vi "Get Tach Period (FPGA).vi"(9 "Threshold Settings":T1={"threshold"=0.0, "hysteresis"=0.0, "slope (rising)"=enum."rising"}, 10 "Max Tach Period (uSec)":u32=1000000, 11 "Analog Tach Signal":fxp<+/-,24,4>) -> (1 "Tach State":T2, 2 "Tach Period (uSec/pulse)":u32)   [LabVIEW 2014, in "Tachometer (SGL).lvlib"]
doc: "Convert analog tachometer signal to RPM"
uses:
  Tachometer (SGL).lvlib
  Tach State.ctl
  Threshold Settings.ctl
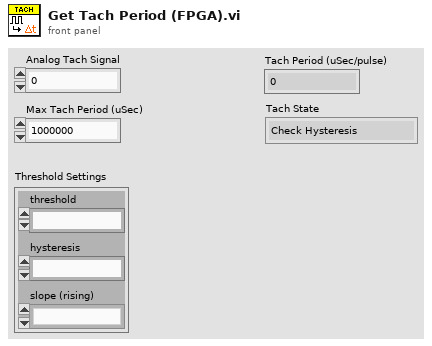
[diagram p1: front panel]
types:
  T1 = typedef "Tachometer (SGL).lvlib/Threshold Settings.ctl" = cluster{"threshold":fxp<+/-,24,4>, "hysteresis":fxp<+/-,24,4>, "slope (rising)":enum16{"falling", "rising"}}
  T2 = typedef "Tachometer (SGL).lvlib/Tach State.ctl" = enum16{"Check Hysteresis", "Check Threshold"}
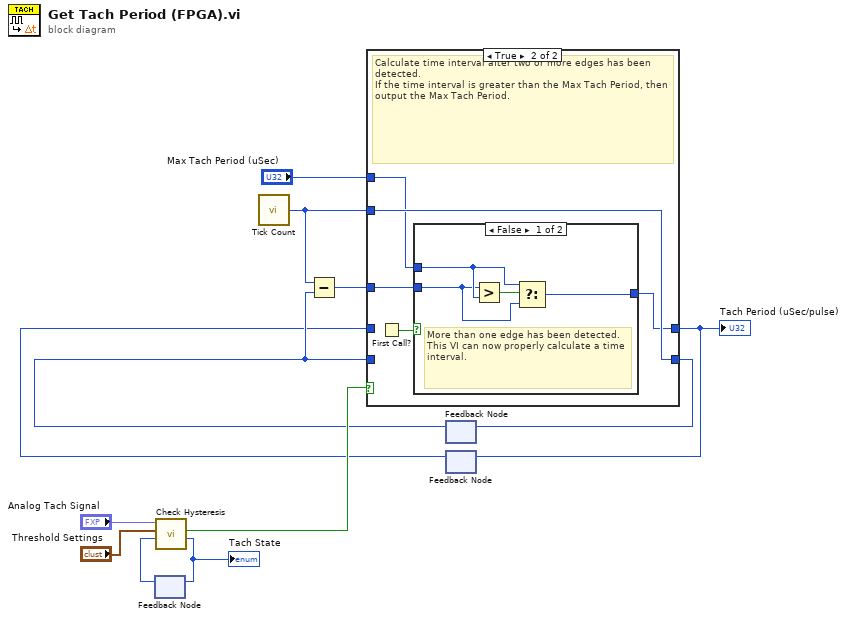
[diagram p0: block diagram]
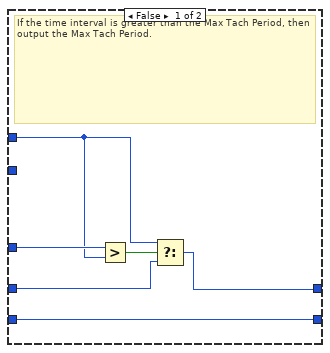
[diagram p2: hidden frame]
diagram:
  n1 = feedback #1() -> (w1:T2)  [unwired: 1 in]
  n2 = call "Check Hysteresis.vi"("State In"=w1, "Threshold Settings"="Threshold Settings", "Analog Tach Signal"="Analog Tach Signal") -> ("State Out"=w2:T2, "Event Occurred?"=w11:bool)  [unwired: 7 in]
  "Tach State" <- w2
  n3 = feedback-in #1(w2) -> ()
  n4 = call "Tick Count"() -> ("Tick Count(uSec)"=w10:u32)
  n5 = feedback #2() -> (w4:u32)  [unwired: 1 in]
  n6 = Subtract(x=w10, y=w4) -> (x-y=w9:u32)
  n7 = feedback #3() -> (w3:u32)  [unwired: 1 in]
  n8 = case shown="True" w11 {
    tunnel: w4 -> [w18 _]
    tunnel: [w18 w23] -> w5
    tunnel: [w13 w20] -> w12
    tunnel: w3 -> [w14 _]
    tunnel: w10 -> [_ w23]
    tunnel: w9 -> [w17 w21]
    tunnel: "Max Tach Period (uSec)" -> [w15 w22]
    frame False {
      # "If the time interval is greater than the Max Tach Period, then output the Max Tach Period."
      n9 = Greater?(x=w17, y=w15) -> (0:w16:bool)
      n10 = Select(t=w15, s=w16, f=w14) -> (s? t:f=w13:u32)
    }
    frame True {
      # "Calculate time interval after two or more edges has been detected.\nIf the time interval is greater than the Max Tach Period, then output the Max Tach Period."
      n11 = First Call?() -> (First Call?: T/F=w19:bool)
      n12 = case shown="False" w19 {
        tunnel: w22 -> [w26 w28]
        tunnel: w21 -> [w25 _]
        tunnel: [w24 w28] -> w20
        frame False {
          # "More than one edge has been detected. This VI can now properly calculate a time interval."
          n13 = Greater?(x=w25, y=w26) -> (0:w27:bool)
          n14 = Select(t=w26, s=w27, f=w25) -> (s? t:f=w24:u32)
        }
        frame True {
          # "Only one edge has been detected, so output the max tach period.  This VI needs two edges to properly calculate a time interval."
        }
      }
    }
  }
  "Tach Period (uSec/pulse)" <- w12
  n15 = feedback-in #2(w5) -> ()
  n16 = feedback-in #3(w12) -> ()
